vi "FGV_ToMessageHandlerEvent.vi"(7 "Command":T1, 8 "error in (no error)":errorcluster) -> (0 "error out":errorcluster, 3 "To message handler event":refnum<user-event>)   [LabVIEW 2011]
uses:
  EnumFgvEventCommand.ctl
  ToMessageHandlerEvent.ctl
  enumMessageCriticity.ctl
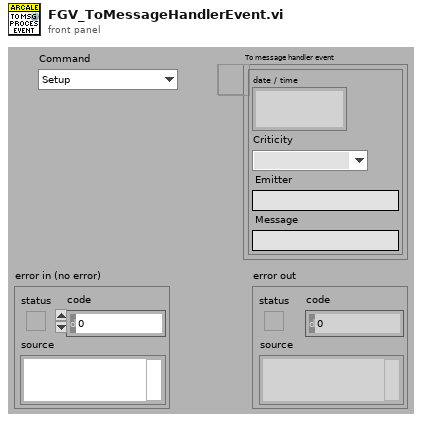
[diagram p1: front panel]
types:
  T1 = typedef "EnumFgvEventCommand.ctl" = enum16{"Setup", "Cleanup", "Get"}
  T2 = typedef "ToMessageHandlerEvent.ctl" = cluster{"date / time":timestamp, "Criticity":T3, "Emitter":string, "Message":string}
  T3 = typedef "enumMessageCriticity.ctl" = enum16{"No error", "Info", "Warning", "Error", "Fatal error"}
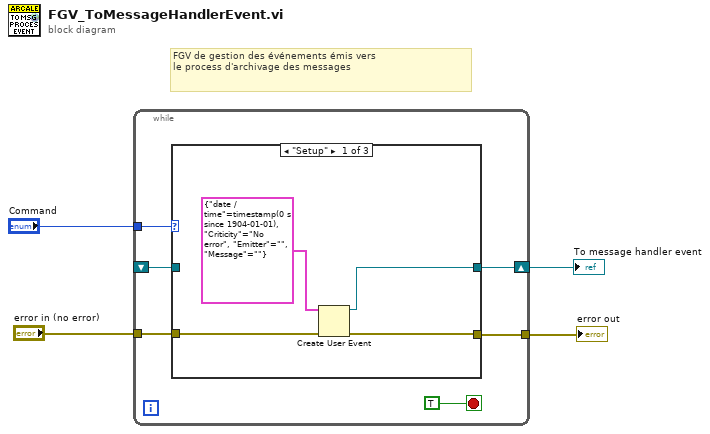
[diagram p0: block diagram]
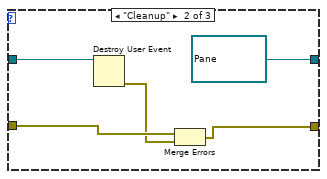
[diagram p2: hidden frame]
diagram:
  # "FGV de gestion des événements émis vers \nle process d'archivage des messages"
  n1 = while {
    tunnel: "error in (no error)" -> [w8]
    tunnel: "Command" -> [w9]
    tunnel: [w7] -> w2
    shift-right: [w6] -> w1
    shift-left: _ -> [w5]
    stop <- TRUE stop-if-true
    n2 = case shown="\"Setup\"" w9 {
      tunnel: w8 -> [w14 w18 w20]
      tunnel: [w12 w16 w20] -> w7
      tunnel: [w11 refnum<user-event> refnum ("To message handler event") w21] -> w6
      tunnel: w5 -> [_ w19 w21]
      frame "Setup" {
        n3 = Create User Event(user event datatype=T2 {"date / time"=timestamp(0 s since 1904-01-01), "Criticity"=enum."No error", "Emitter"="", "Message"=""} ("To message handler event"), error in=w14) -> (user event=w11:refnum<user-event>, error out=w12:errorcluster)
      }
      frame "Cleanup" {
        n4 = Destroy User Event(user event=w19) -> (error out=w17:errorcluster)  [unwired: 1 in]
        n5 = Merge Errors(w18, w17) -> (w16:errorcluster)
      }
      frame "Get" {
      }
    }
  }
  "error out" <- w2
  "To message handler event" <- w1
